vi "Read Controller Details.vi"(8 "error in (no error)":errorcluster, 9 "Plugin File Path":path, 10 "Plugin Details in":T2, 11 "Refnum in":T1) -> (0 "error out":errorcluster, 2 "Plugin Details out":T2, 3 "refnum out":T1)   [LabVIEW 2020, in "RxnRover.lvlib" / "Plugin Manager.lvlib"]
uses:
  Plugin Manager.lvlib
  Plugin Details.ctl
  Plugin Servers/Controller/Controller Type.ctl
  Plugin Types.ctl
  Config Error.ctl
  <vilib>/Utility/config.llb/Config Data RefNum.ctl
  <vilib>/Utility/config.llb/Read Key (String).vi
  <vilib>/Utility/config.llb/Read Key (Path).vi
  <vilib>/Utility/config.llb/NI_LVConfig.lvlib
  Plugin Servers/Controller/Generic Plugin.lvclass
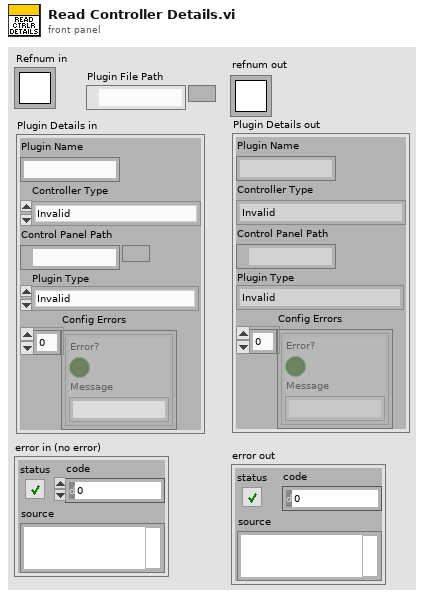
[diagram p1: front panel]
types:
  T1 = typedef "NI_LVConfig.lvlib/Config Data RefNum.ctl" = refnum<k1>
  T2 = typedef "RxnRover.lvlib/Plugin Manager.lvlib/Plugin Details.ctl" = cluster{"Plugin Name":string, "Controller Type":T3, "Control Panel Path":path, "Plugin Type":T4, "Config Errors":T5[]}
  T3 = typedef "RxnRover.lvlib/Generic Plugin.lvclass/Controller Type.ctl" = enum16{"Invalid", "Temperature Controller", "Pump Controller", "Syringe Pump", "Generic Optimizer", "LC Parser"}
  T4 = typedef "RxnRover.lvlib/Plugin Manager.lvlib/Plugin Types.ctl" = enum16{"Invalid", "Optimizer", "Analyzer", "Hardware"}
  T5 = typedef "RxnRover.lvlib/Plugin Manager.lvlib/Config Error.ctl" = cluster{"Error?":bool, "Message":string}
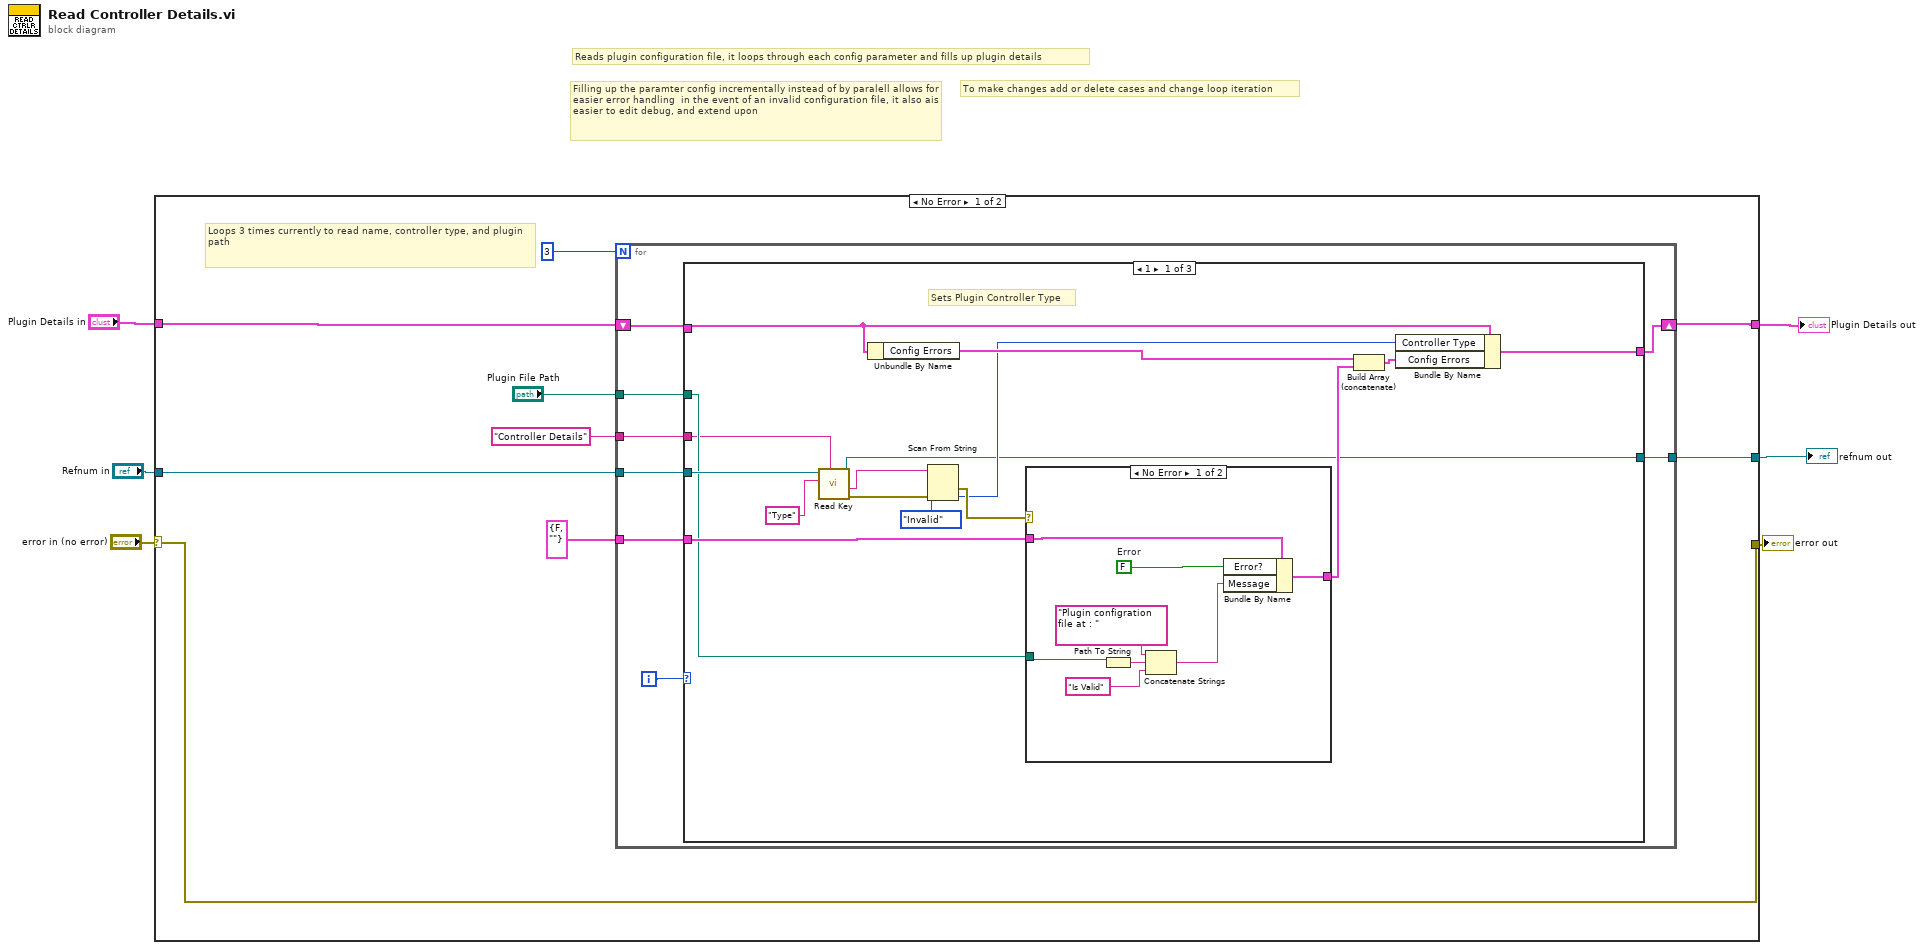
[diagram p0: block diagram]
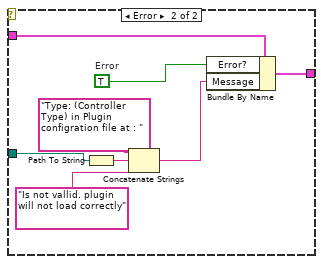
[diagram p2: hidden frame]
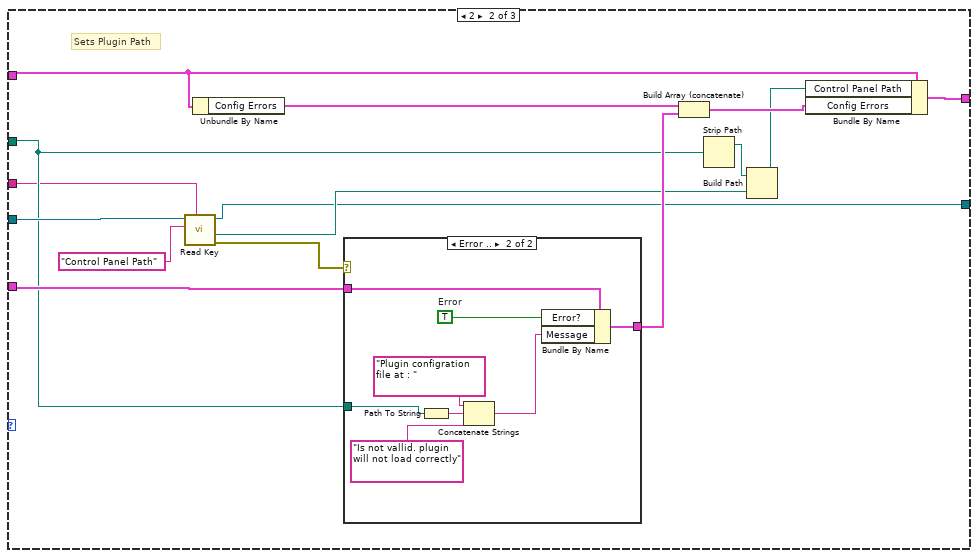
[diagram p3: hidden frame]
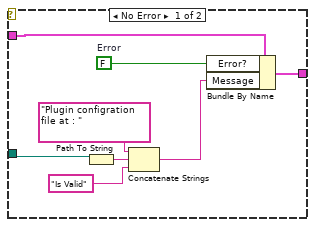
[diagram p4: hidden frame]
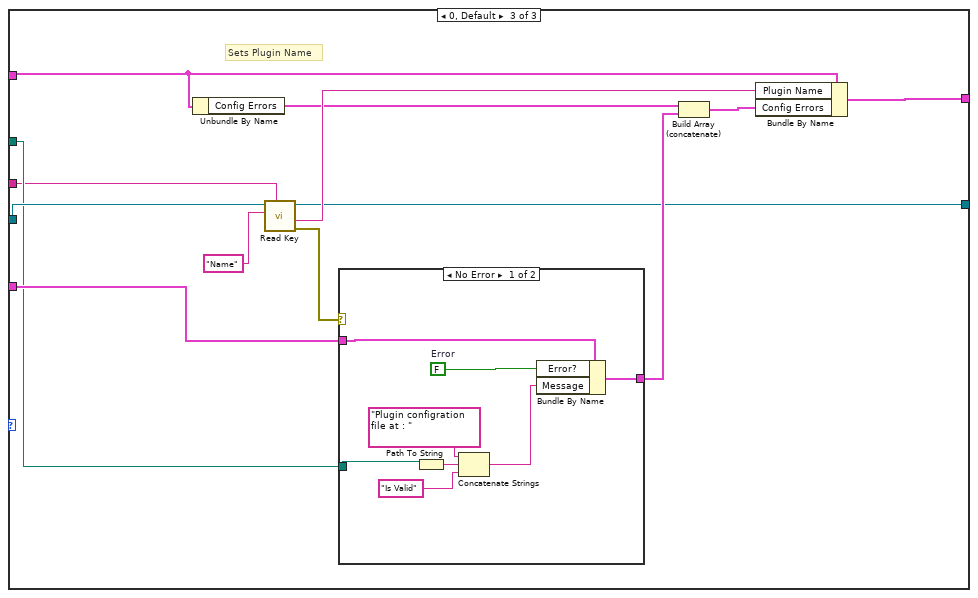
[diagram p5: hidden frame]
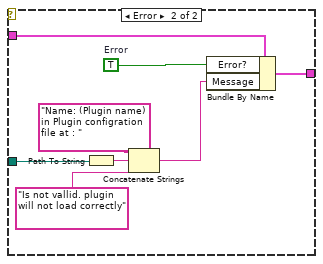
[diagram p6: hidden frame]
diagram:
  # "To make changes add or delete cases and change loop iteration"
  # "Filling up the paramter config incrementally instead of by paralell allows for easier error handling  in the event of an invalid configuration file, it also ais easier to edit debug, and extend upon"
  # "Reads plugin configuration file, it loops through each config parameter and fills up plugin details"
  n1 = case shown="No Error" "error in (no error)" {
    selector: "error in (no error)" -> [w8 w118]
    tunnel: "Plugin Details in" -> [w13 w116]
    tunnel: [w10 w116] -> w5
    tunnel: [w8 w118] -> w4
    tunnel: [w9 w117] -> w3
    tunnel: "Refnum in" -> [w12 w117]
    frame No Error {
      # "Loops 3 times currently to read name, controller type, and plugin path"
      n2 = for {
        N: 3 -> [_]
        tunnel: T5 {"Error?"=FALSE, "Message"=""} ("Config Error") -> [w22]
        tunnel: w12 -> [w20]
        tunnel: "Plugin File Path" -> [w19]
        tunnel: [w17] -> w9
        tunnel: "Controller Details" -> [w16]
        shift-right: [w18] -> w10
        shift-left: w13 -> [w23]
        i -> [w21]
        n3 = case shown="1" w21 {
          tunnel: w23 -> [w37 w67 w95]
          tunnel: w22 -> [w38 w68 w96]
          tunnel: [w28 w63 w91] -> w18
          tunnel: w20 -> [w27 w59 w90]
          tunnel: w19 -> [w26 w58 w89]
          tunnel: [w25 w57 w88] -> w17
          tunnel: w16 -> [w24 w56 w87]
          frame 1 {
            # "Sets Plugin Controller Type"
            n4 = call-poly <vilib>:"Read Key.vi"("section"=w24, "key"="Type", "refnum"=w27) -> ("error out"=w32:errorcluster, "value"=w30:string, "refnum out"=w25:T1)  [unwired: 5 in, 1 out]
            n5 = Unbundle By Name(w37) -> ("Config Errors"=w35:T5[])
            n6 = Scan From String(input string=w30, error in=w32, default 1=Controller_Type."Invalid" ("Controller Type")) -> (error out=w31:errorcluster, output 1=w29:T3)  [unwired: 2 in, 2 out]
            n7 = case shown="No Error" w31 {
              tunnel: w26 -> [w47 w49]
              tunnel: w38 -> [w43 w50]
              tunnel: [w40 w51] -> w36
              frame No Error {
                w42 = FALSE  # Error
                n8 = Path To String(path=w47) -> (string=w46:string)
                n9 = Concatenate Strings("Plugin configration file at : ", w46, "Is Valid") -> (w41:string)
                n10 = Bundle By Name(cluster=w43, "Error?"=w42, "Message"=w41) -> (w40:T5)
              }
              frame Error {
                w53 = TRUE  # Error
                n11 = Path To String(path=w49) -> (string=w55:string)
                n12 = Concatenate Strings("Type: (Controller Type) in Plugin configration file at : ", w55, "Is not vallid. plugin will not load correctly") -> (w52:string)
                n13 = Bundle By Name(cluster=w50, "Error?"=w53, "Message"=w52) -> (w51:T5)
              }
            }
            n14 = Build Array (concatenate)(w35, w36) -> (w34:T5[])
            n15 = Bundle By Name(cluster=w37, "Controller Type"=w29, "Config Errors"=w34) -> (w28:T2)
          }
          frame 2 {
            # "Sets Plugin Path"
            n16 = call-poly <vilib>:"Read Key.vi"("section"=w56, "key"="Control Panel Path", "refnum"=w59) -> ("error out"=w69:errorcluster, "value"=w60:path, "refnum out"=w57:T1)  [unwired: 5 in, 1 out]
            n17 = Unbundle By Name(w67) -> ("Config Errors"=w65:T5[])
            n18 = case shown="Error .." w69 {
              tunnel: w58 -> [w78 w80]
              tunnel: w68 -> [w74 w81]
              tunnel: [w71 w82] -> w66
              frame No Error {
                w73 = FALSE  # Error
                n19 = Path To String(path=w78) -> (string=w77:string)
                n20 = Concatenate Strings("Plugin configration file at : ", w77, "Is Valid") -> (w72:string)
                n21 = Bundle By Name(cluster=w74, "Error?"=w73, "Message"=w72) -> (w71:T5)
              }
              frame Error {
                w84 = TRUE  # Error
                n22 = Path To String(path=w80) -> (string=w86:string)
                n23 = Concatenate Strings("Plugin configration file at : ", w86, "Is not vallid. plugin will not load correctly") -> (w83:string)
                n24 = Bundle By Name(cluster=w81, "Error?"=w84, "Message"=w83) -> (w82:T5)
              }
            }
            n25 = Build Array (concatenate)(w65, w66) -> (w64:T5[])
            n26 = Strip Path(path=w58) -> (stripped path=w62:path)  [unwired: 1 out]
            n27 = Build Path(base path=w62, name or relative path=w60) -> (appended path=w61:path)
            n28 = Bundle By Name(cluster=w67, "Control Panel Path"=w61, "Config Errors"=w64) -> (w63:T2)
          }
          frame 0, Default {
            # "Sets Plugin Name"
            n29 = Unbundle By Name(w95) -> ("Config Errors"=w93:T5[])
            n30 = call-poly <vilib>:"Read Key.vi"("section"=w87, "key"="Name", "refnum"=w90) -> ("error out"=w97:errorcluster, "value"=w98:string, "refnum out"=w88:T1)  [unwired: 5 in, 1 out]
            n31 = case shown="No Error" w97 {
              tunnel: w89 -> [w107 w108]
              tunnel: w96 -> [w103 w110]
              tunnel: [w100 w111] -> w94
              frame No Error {
                w102 = FALSE  # Error
                n32 = Path To String(path=w107) -> (string=w106:string)
                n33 = Concatenate Strings("Plugin configration file at : ", w106, "Is Valid") -> (w101:string)
                n34 = Bundle By Name(cluster=w103, "Error?"=w102, "Message"=w101) -> (w100:T5)
              }
              frame Error {
                w113 = TRUE  # Error
                n35 = Path To String(path=w108) -> (string=w115:string)
                n36 = Concatenate Strings("Name: (Plugin name) in Plugin configration file at : ", w115, "Is not vallid. plugin will not load correctly") -> (w112:string)
                n37 = Bundle By Name(cluster=w110, "Error?"=w113, "Message"=w112) -> (w111:T5)
              }
            }
            n38 = Build Array (concatenate)(w93, w94) -> (w92:T5[])
            n39 = Bundle By Name(cluster=w95, "Plugin Name"=w98, "Config Errors"=w92) -> (w91:T2)
          }
        }
      }
    }
    frame Error {
    }
  }
  "Plugin Details out" <- w5
  "error out" <- w4
  "refnum out" <- w3
